vi "Set Aircraft Mode.vi"(8 "Error In":errorcluster, 11 "Aircraft Mode":T1=enum."LOITER") -> (0 "error out":errorcluster, 3 "Selected Aircraft ID Out":u8)   [LabVIEW 2014]
uses:
  Controls/MAVLink Flight modes.ctl
  Aircraft Information/Sub VI/Selected Aircraft/SubVI/Get Selected Aircraft.vi
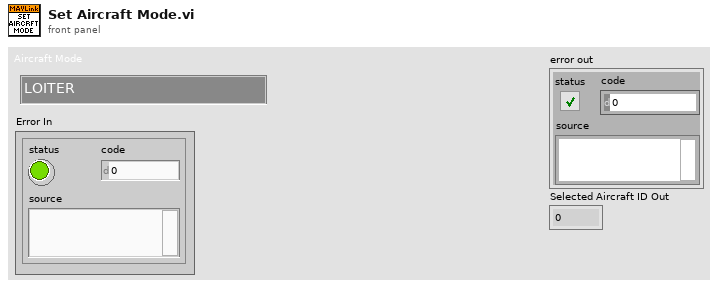
[diagram p1: front panel]
types:
  T1 = typedef "MAVLink Flight modes.ctl" = enum32{"STABILISE", "ACRO", "ALT HOLD", "AUTO", "GUIDED", "LOITER", "RTL", "CIRCLE", "UNKNOWN1", "LAND", "OF LOITER", "DRIFT", "UNKNOWN2", "SPORT", "FLIP", "AUTO TUNE", "POS HOLD", "BRAKE"}
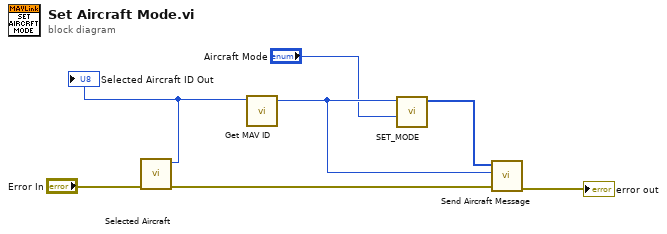
[diagram p0: block diagram]
diagram:
  n1 = call-poly "Selected Aircraft.vi"("Error In"="Error In") -> ("Error Out"=w3:errorcluster, "Selected Aircraft ID Out"=w5:u8)  [unwired: 9 in]
  "Selected Aircraft ID Out" <- w5
  n2 = call "Get MAV ID.vi"("Aircraft Index"=w5) -> ("Aircraft ID"=w6:u8)  [unwired: 9 in, 1 out]
  n3 = call "SET_MODE.vi"("Flight Mode"="Aircraft Mode", "target_system"=w6) -> ("MAVLink Message"=w7:u8[])  [unwired: 9 in]
  n4 = call "Send Aircraft Message.vi"("error in (no error)"=w3, "Aircraft ID"=w6, "MAVLink Message"=w7) -> ("error out"=→"error out":errorcluster)  [unwired: 8 in]
